vi "ScratchTest.vi"() -> ()   [LabVIEW 2014]
panel:
  in  "stop":bool
  out "lo(x) 3":u8
  out "hi(x) 3":u8
  out "lo(x) 2":u8
  out "hi(x) 2":u8
  out "unsigned 32bit integer":u32
  out "lo(x)":u8
  out "hi(x)":u8
  in  "U16":u16
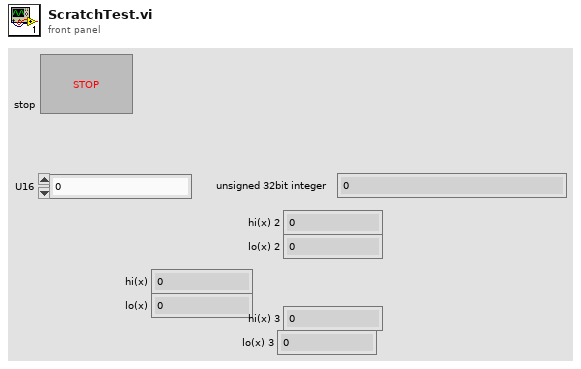
[diagram p1: front panel]
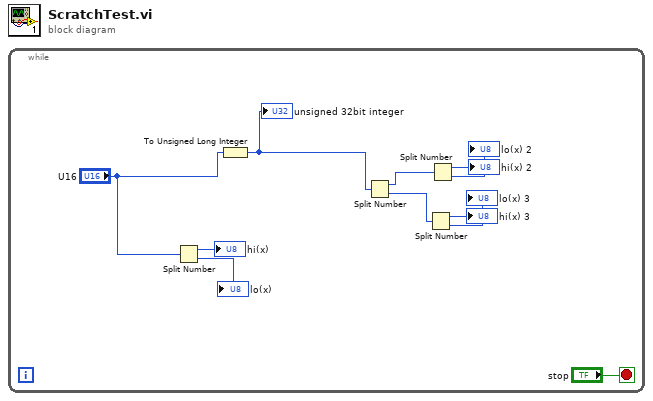
[diagram p0: block diagram]
diagram:
  n1 = while {
    stop <- "stop" stop-if-true
    n2 = Split Number(x="U16") -> (hi(x)=→"hi(x)":u8, lo(x)=→"lo(x)":u8)
    n3 = To Unsigned Long Integer(number="U16") -> (unsigned 32bit integer=w8:u32)
    "unsigned 32bit integer" <- w8
    n4 = Split Number(x=w8) -> (hi(x)=w7:u16, lo(x)=w6:u16)
    n5 = Split Number(x=w6) -> (hi(x)=→"hi(x) 3":u8, lo(x)=→"lo(x) 3":u8)
    n6 = Split Number(x=w7) -> (hi(x)=→"hi(x) 2":u8, lo(x)=→"lo(x) 2":u8)
  }
